vi "inherrited settings.vi"(8 "Measurement Type In":T1, 9 "Sphere Indicator In":T3, 10 "Base Path In":path, 11 "Inherrit Settings Command":T2) -> (0 "Measurement Type Out":T1, 1 "Sphere Indicator out":T3, 3 "Base Path out":path)   [LabVIEW 2014, in "AvaSpec.lvlib"]
uses:
  AvaSpec.lvlib
  Acquisition/Sphere Indicator.ctl
  controls/inherrited settings command.ctl
  Settings/Measurement Type.ctl
  Acquisition/AvaSpec Acquisition.lvlib
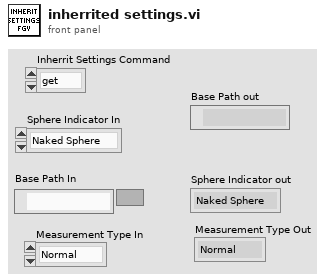
[diagram p1: front panel]
types:
  T1 = typedef "AvaSpec.lvlib/AvaSpec Acquisition.lvlib/Measurement Type.ctl" = enum16{"Normal", "Calibration", "Dark"}
  T2 = typedef "AvaSpec.lvlib/inherrited settings command.ctl" = enum16{"get", "set"}
  T3 = typedef "AvaSpec.lvlib/Sphere Indicator.ctl" = enum16{"Naked Sphere", "Insulated Sphere"}
  T4 = cluster{"Base Path In":path, "Measurement Type In":T1, "Sphere Indicator In":T3}
  T5 = cluster{"Base Path In":path, "Measurement Type In":T1, "Sphere Indicator In":T3}[]
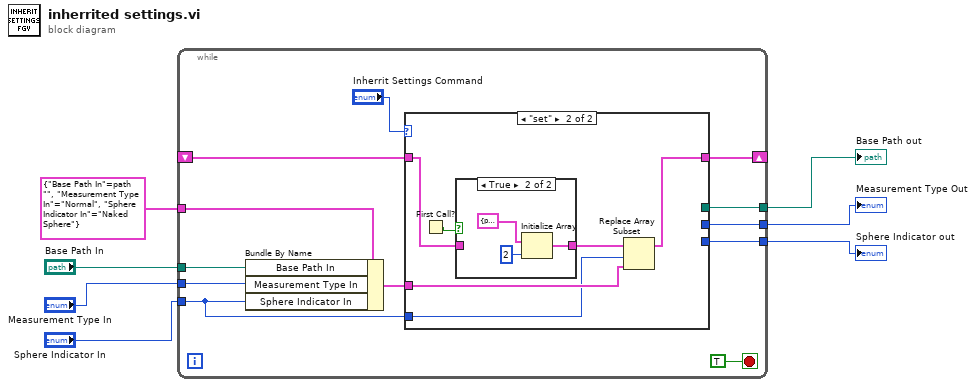
[diagram p0: block diagram]
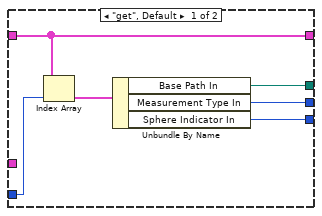
[diagram p2: hidden frame]
diagram:
  n1 = while {
    tunnel: "Base Path In" -> [w14]
    tunnel: "Sphere Indicator In" -> [w11]
    shift-right: [w18] -> _
    shift-left: _ -> [w17]
    tunnel: "Measurement Type In" -> [w13]
    tunnel: T4 {"Base Path In"=path "", "Measurement Type In"=enum."Normal", "Sphere Indicator In"=enum."Naked Sphere"} -> [w15]
    tunnel: [w10] -> w4
    tunnel: [w9] -> w3
    tunnel: [w8] -> w2
    stop <- TRUE stop-if-true
    n2 = Bundle By Name(cluster=w15, "Base Path In"=w14, "Measurement Type In"=w13, "Sphere Indicator In"=w11) -> (w12:T4)
    n3 = case shown="\"set\"" "Inherrit Settings Command" {
      tunnel: [w24 w26] -> w18
      tunnel: w17 -> [w24 w31]
      tunnel: w12 -> [_ w28]
      tunnel: w11 -> [w25 w27]
      tunnel: [w22 _] -> w10
      tunnel: [w21 _] -> w9
      tunnel: [w20 _] -> w8
      frame "get", Default {
        n4 = Index Array(array=w24, index=w25) -> (element=w23:T4)
        n5 = Unbundle By Name(w23) -> ("Base Path In"=w22:path, "Measurement Type In"=w21:T1, "Sphere Indicator In"=w20:T3)
      }
      frame "set" {
        n6 = First Call?() -> (First Call?: T/F=w30:bool)
        n7 = case shown="True" w30 {
          tunnel: [w32 w33] -> w29
          tunnel: w31 -> [w32 _]
          frame False {
          }
          frame True {
            n8 = Initialize Array(T4 {"Base Path In"=path "", "Measurement Type In"=enum."Normal", "Sphere Indicator In"=enum."Naked Sphere"}, 2 ("dimension size")) -> (w33:T5)
          }
        }
        n9 = Replace Array Subset(array=w29, new element=w28, index=w27) -> (w26:T5)
      }
    }
  }
  "Base Path out" <- w4
  "Sphere Indicator out" <- w2
  "Measurement Type Out" <- w3
